vi "Init.vi"(8 "error in (no error)":errorcluster, 10 "Instrument String":variant, 11 "Hioki BT4560B":refnum<class "Hioki BT4560B.lvclass">) -> (0 "error out":errorcluster, 2 "Found?":bool=TRUE, 3 "Hioki BT4560B out":refnum<class "Hioki BT4560B.lvclass">)   [LabVIEW 2025, in "ACIR.lvlib" / "Hioki BT4560B.lvclass"]
uses:
  Hioki BT4560B.lvclass
  ACIR configuration/ACIR configuration.lvclass
  Hioki BT4560B.lvclass/Hioki BT4560B.ctl
  Users/Public/Documents/Sandia National Labs/TSS Plugin/Abstract Engine.lvlibp/Plugin/Abstract/Instrument configuration/Read Instrument Setting.vi
  Users/Public/Documents/Sandia National Labs/TSS Plugin/CEF.lvlibp/serializable configuration/CEF_serializable configuration.lvclass
  <instrlib>/HIOKI BT4560/HIOKI BT4560.lvlib
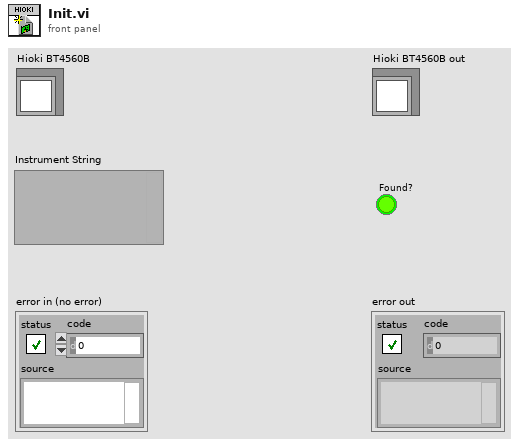
[diagram p1: front panel]
types:
  T1 = typedef "Abstract Engine.lvlibp/Instrument configuration.lvclass/Default Instrument.ctl" = cluster{"Type":string, "Address":string, "SW Alias":string, "Description":string, "Enabled":bool}
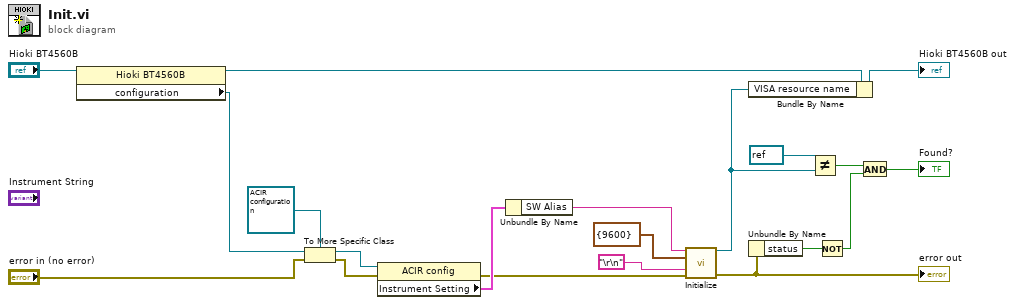
[diagram p0: block diagram]
diagram:
  n1 = property class="Hioki BT4560B"(reference="Hioki BT4560B") -> (reference out=w18:refnum<class "Hioki BT4560B.lvclass">, "configuration"=w11:refnum<class "CEF_serializable configuration.lvclass">)  [unwired: 1 in, 1 out]
  n2 = To More Specific Class(target class=refnum<class "ACIR configuration.lvclass"> refnum ("ACIR.lvlib:ACIR config"), reference=w11, error in="error in (no error)") -> (specific class reference=w12:refnum<class "ACIR configuration.lvclass">, error out=w13:errorcluster)
  n3 = property class="ACIR config"(reference=w12, error in=w13) -> (error out=w5:errorcluster, "Instrument Setting"=w8:T1)  [unwired: 1 out]
  n4 = Unbundle By Name(w8) -> ("SW Alias"=w4:string)
  n5 = call <instrlib>:"Initialize.vi"("VISA resource name"=w4, "Serial Configuration"=cluster{"Baud Rate":u32} {"Baud Rate"=9600} ("Configuration"), "Terminator"="\r\n", "error in (no error)"=w5) -> ("VISA resource name out"=w2:refnum<visa-resource-name>, "error out"=w3:errorcluster)  [unwired: 9 in, 1 out]
  "error out" <- w3
  n6 = Bundle By Name(cluster=w18, "VISA resource name"=w2) -> (→"Hioki BT4560B out":refnum<class "Hioki BT4560B.lvclass">)
  n7 = Unbundle By Name(w3) -> ("status"=w17:bool)
  n8 = Not Equal?(x=refnum<visa-resource-name> refnum ("VISA resource name out"), y=w2) -> (x != y?=w15:bool)
  n9 = Not(x=w17) -> (.not. x?=w16:bool)
  n10 = And(x=w15, y=w16) -> (x .and. y?=→"Found?":bool)
